vi "read Kin v2.vi"(7 "file path":path) -> (0 "sensor 3 rotation":dbl[][](array[numeric]), 1 "sensor 1 rotation":dbl[][](array[numeric]), 2 "sensor 2 acceleration":dbl[][](array[numeric]), 3 "sensor 1 acceleration":dbl[][](array[numeric]), 4 "sensor 3 acceleration":dbl[][](array[numeric]), 5 "Frequency (Hz)":dbl, 6 "sensor 2 rotation":dbl[][](array[numeric]))   [LabVIEW 2009]
uses:
  <vilib>/Utility/file.llb/Read From Spreadsheet File (DBL).vi
panel:
  out "event":dbl[](array[numeric])
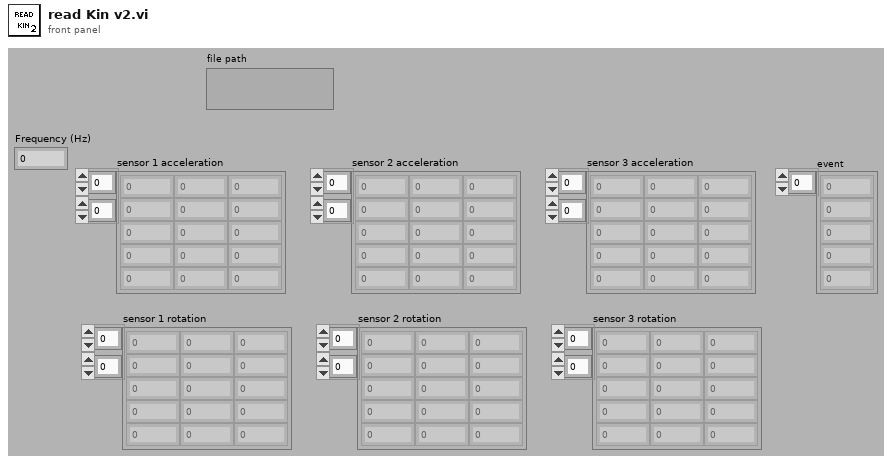
[diagram p1: front panel]
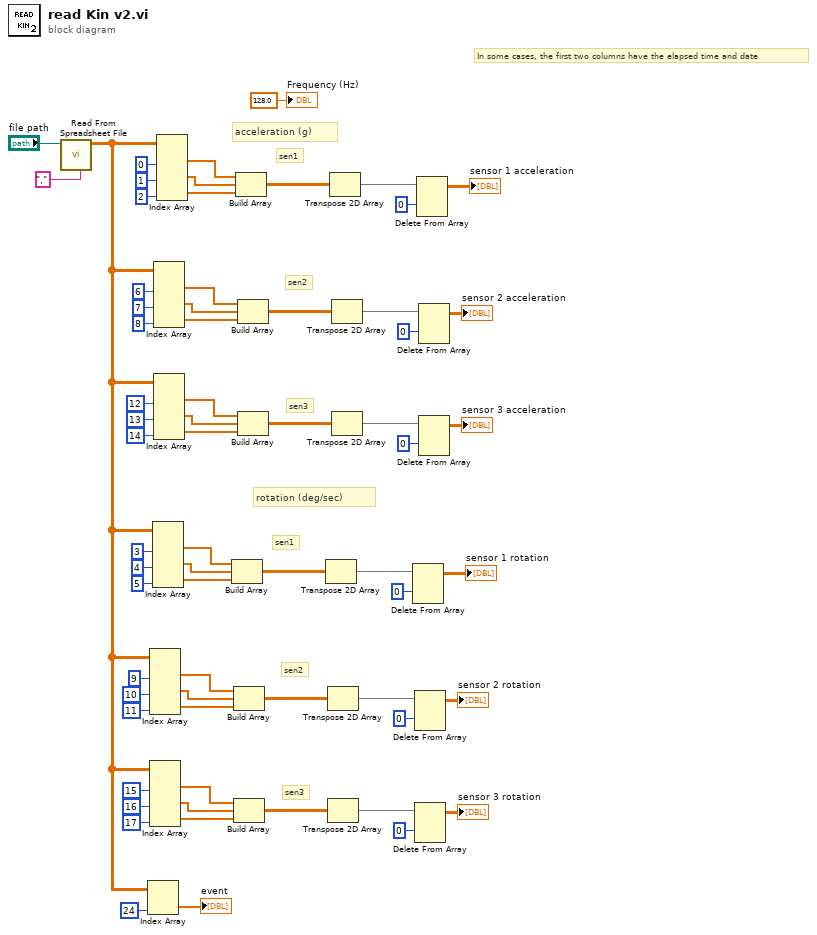
[diagram p0: block diagram]
diagram:
  # "In some cases, the first two columns have the elapsed time and date"
  # "sen3"
  # "sen2"
  # "sen1"
  # "rotation (deg/sec)"
  # "sen3"
  # "sen2"
  # "sen1"
  # "acceleration (g)"
  n1 = call-poly <vilib>:"Read From Spreadsheet File.vi"("delimiter (\\t)"="," ("delimiter (\\t)"), "file path (dialog if empty)"="file path") -> ("all rows"=w7:dbl[][])  [unwired: 5 in, 4 out]
  n2 = Index Array(array=w7, index (col)=24 ("disabled index (col)")) -> (element=→"event":dbl[])  [unwired: 1 in]
  n3 = Index Array(array=w7, index (col) #1=9 ("disabled index (col)"), index (col) #2=10 ("index (col)"), index (col) #3=11 ("index (col)")) -> (element #1=w21:dbl[], element #2=w22:dbl[], element #3=w23:dbl[])  [unwired: 3 in]
  n4 = Index Array(array=w7, index (col) #1=15 ("disabled index (col)"), index (col) #2=16 ("index (col)"), index (col) #3=17 ("index (col)")) -> (element #1=w11:dbl[], element #2=w12:dbl[], element #3=w13:dbl[])  [unwired: 3 in]
  n5 = Index Array(array=w7, index (col) #1=3 ("disabled index (col)"), index (col) #2=4 ("index (col)"), index (col) #3=5 ("index (col)")) -> (element #1=w35:dbl[], element #2=w34:dbl[], element #3=w33:dbl[])  [unwired: 3 in]
  n6 = Index Array(array=w7, index (col) #1=6 ("disabled index (col)"), index (col) #2=7 ("index (col)"), index (col) #3=8 ("index (col)")) -> (element #1=w3:dbl[], element #2=w2:dbl[], element #3=w51:dbl[])  [unwired: 3 in]
  n7 = Index Array(array=w7, index (col) #1=12 ("disabled index (col)"), index (col) #2=13 ("index (col)"), index (col) #3=14 ("index (col)")) -> (element #1=w42:dbl[], element #2=w43:dbl[], element #3=w44:dbl[])  [unwired: 3 in]
  n8 = Index Array(array=w7, index (col) #1=0 ("disabled index (col)"), index (col) #2=1 ("index (col)"), index (col) #3=2 ("index (col)")) -> (element #1=w1:dbl[], element #2=w62:dbl[], element #3=w61:dbl[])  [unwired: 3 in]
  n9 = Build Array(w35, w34, w33) -> (w32:dbl[][])
  n10 = Build Array(w21, w22, w23) -> (w26:dbl[][])
  n11 = Build Array(w11, w12, w13) -> (w16:dbl[][])
  n12 = Build Array(w1, w62, w61) -> (w60:dbl[][])
  n13 = Build Array(w3, w2, w51) -> (w54:dbl[][])
  n14 = Build Array(w42, w43, w44) -> (w47:dbl[][])
  n15 = Transpose 2D Array(2D array=w32) -> (transposed array=w31:dbl[][])
  n16 = Transpose 2D Array(2D array=w26) -> (transposed array=w25:dbl[][])
  n17 = Transpose 2D Array(2D array=w16) -> (transposed array=w15:dbl[][])
  n18 = Transpose 2D Array(2D array=w60) -> (transposed array=w59:dbl[][])
  n19 = Transpose 2D Array(2D array=w54) -> (transposed array=w53:dbl[][])
  n20 = Transpose 2D Array(2D array=w47) -> (transposed array=w46:dbl[][])
  n21 = Delete From Array(array=w31, index (row)=0) -> (array with subset deleted=→"sensor 1 rotation":dbl[][])  [unwired: 2 in, 1 out]
  n22 = Delete From Array(array=w25, index (row)=0) -> (array with subset deleted=→"sensor 2 rotation":dbl[][])  [unwired: 2 in, 1 out]
  n23 = Delete From Array(array=w15, index (row)=0) -> (array with subset deleted=→"sensor 3 rotation":dbl[][])  [unwired: 2 in, 1 out]
  n24 = Delete From Array(array=w59, index (row)=0) -> (array with subset deleted=→"sensor 1 acceleration":dbl[][])  [unwired: 2 in, 1 out]
  n25 = Delete From Array(array=w53, index (row)=0) -> (array with subset deleted=→"sensor 2 acceleration":dbl[][])  [unwired: 2 in, 1 out]
  n26 = Delete From Array(array=w46, index (row)=0) -> (array with subset deleted=→"sensor 3 acceleration":dbl[][])  [unwired: 2 in, 1 out]
  "Frequency (Hz)" <- 128.0 ("Frequency (Hz)")
